vi "GenAndWrite.vi"(8 "error in (no error)":errorcluster, 9 "Prompt?":bool=TRUE caption="Prompt for overwrite? (T)", 10 "Path":path, 11 "Config":T1) -> (0 "error out":errorcluster)   [LabVIEW 2020]
uses:
  <vilib>/WebServerConfig/Config.ctl
  <vilib>/WebServerConfig/Server.ctl
  <vilib>/WebServerConfig/Alias.ctl
  <vilib>/WebServerConfig/ErrorDocument.ctl
  <vilib>/WebServerConfig/Action.ctl
  <vilib>/WebServerConfig/Redirect.ctl
  <vilib>/WebServerConfig/Interface.ctl
  <vilib>/WebServerConfig/AddHandler.ctl
  <vilib>/WebServerConfig/SSL.ctl
  <vilib>/WebServerConfig/CustomLog.ctl
  <vilib>/WebServerConfig/LoadModule.ctl
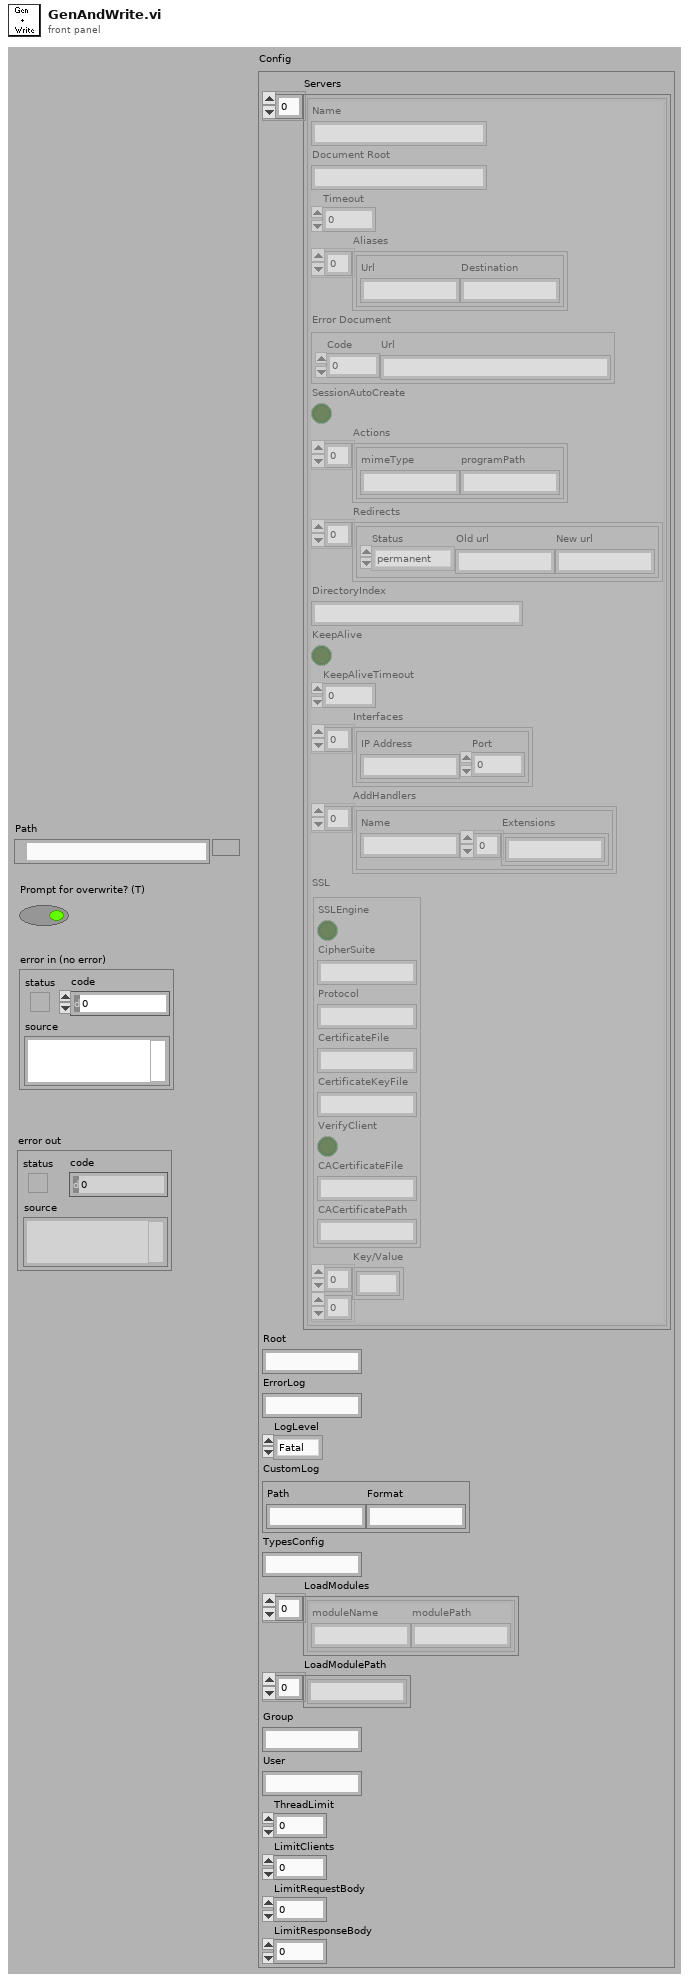
[diagram p1: front panel]
types:
  T1 = typedef "Config.ctl" = cluster{"Servers":T2[], "Root":string, "ErrorLog":string, "LogLevel":enum16{"Fatal", "Error", "Warn", "Info", "Debug", "5", "6", "7", "8", "Verbose"}, "CustomLog":T10, "TypesConfig":string, "LoadModules":T11[], "LoadModulePath":string[], "Group":string, "User":string, "ThreadLimit":u32, "LimitClients":u32, "LimitRequestBody":u32, "LimitResponseBody":u32}
  T2 = typedef "Server.ctl" = cluster{"Name":string, "Document Root":string, "Timeout":u32, "Aliases":T3[], "Error Document":T4, "SessionAutoCreate":bool, "Actions":T5[], "Redirects":T6[], "DirectoryIndex":string, "KeepAlive":bool, "KeepAliveTimeout":u32, "Interfaces":T7[], "AddHandlers":T8[], "SSL":T9, "Key/Value":string[][]}
  T3 = typedef "Alias.ctl" = cluster{"Url":string, "Destination":string}
  T4 = typedef "ErrorDocument.ctl" = cluster{"Code":u16, "Url":string}
  T5 = typedef "Action.ctl" = cluster{"mimeType":string, "programPath":string}
  T6 = typedef "Redirect.ctl" = cluster{"Status":enum16{"permanent", "temp", "seeother", "gone"}, "Old url":string, "New url":string}
  T7 = typedef "Interface.ctl" = cluster{"IP Address":string, "Port":u16}
  T8 = typedef "AddHandler.ctl" = cluster{"Name":string, "Extensions":string[]}
  T9 = typedef "SSL.ctl" = cluster{"SSLEngine":bool, "CipherSuite":string, "Protocol":string, "CertificateFile":string, "CertificateKeyFile":string, "VerifyClient":bool, "CACertificateFile":string, "CACertificatePath":string}
  T10 = typedef "CustomLog.ctl" = cluster{"Path":string, "Format":string}
  T11 = typedef "LoadModule.ctl" = cluster{"moduleName":string, "modulePath":string}
  T12 = enum16{"open", "replace", "create", "open or create", "replace or create", "replace or create with confirmation"}
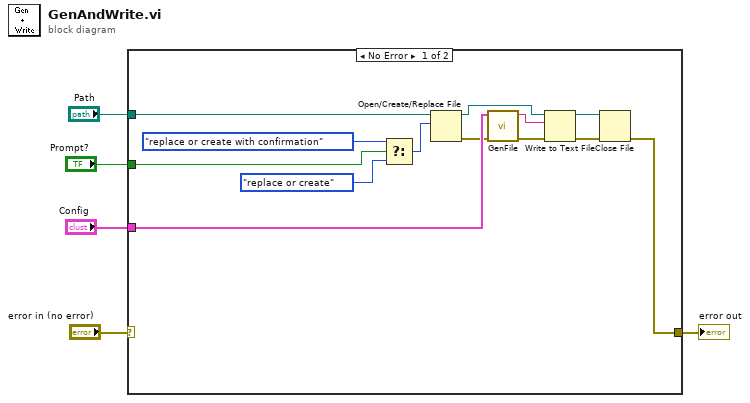
[diagram p0: block diagram]
diagram:
  n1 = case shown="No Error" "error in (no error)" {
    selector: "error in (no error)" -> [_ w19]
    tunnel: [w10 w19] -> w4
    tunnel: "Path" -> [w18 _]
    tunnel: "Config" -> [w17 _]
    tunnel: "Prompt?" -> [w7 _]
    frame No Error {
      n2 = Select(t=T12."replace or create with confirmation" ("operation (0:open)"), s=w7, f=T12."replace or create") -> (s? t:f=w9:T12)
      n3 = Open/Create/Replace File(file path (use dialog)=w18, operation (0:open)=w9) -> (refnum out=w14:refnum<file>, error out=w16:errorcluster)  [unwired: 4 in, 1 out]
      n4 = call <vilib>:"GenFile.vi"("error in"=w16, "Config"=w17) -> ("error out"=w15:errorcluster, "FileContents"=w13:string)  [unwired: 8 in]
      n5 = Write to Text File(file (use dialog)=w14, text=w13, error in=w15) -> (refnum out=w11:refnum<file>, error out=w12:errorcluster)  [unwired: 1 in, 1 out]
      n6 = Close File(refnum=w11, error in=w12) -> (error out=w10:errorcluster)  [unwired: 1 out]
    }
    frame Error {
    }
  }
  "error out" <- w4
